vi "OpenG Dictionary.vi"() -> ()   [LabVIEW 2013]
uses:
  <userlib>/_OpenG.lib/dictionary/dictionary.llb/Dictionary Update (by scalar value)__ogtk.vi
panel:
  out "get value":variant
  in  "key":string
  in  "Get Value":bool
  out "item poped":cluster{"key":variant, "value":variant}
  in  "Pop":bool
  in  "item to be added":cluster{"key":string, "Value":dbl}
  in  "Add":bool
  out "items":cluster{"key":variant, "value":variant}[](array[cluster])
  out "Dict size":i32
  in  "stop":bool
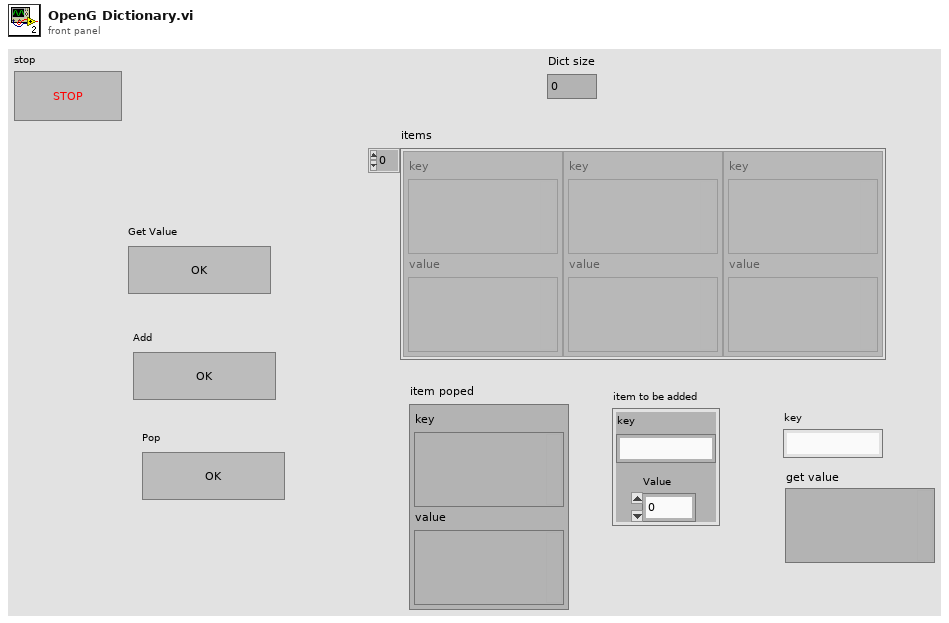
[diagram p1: front panel]
types:
  T1 = typedef "Dictionary Object RefNum__ogtk.ctl" = refnum<k1>
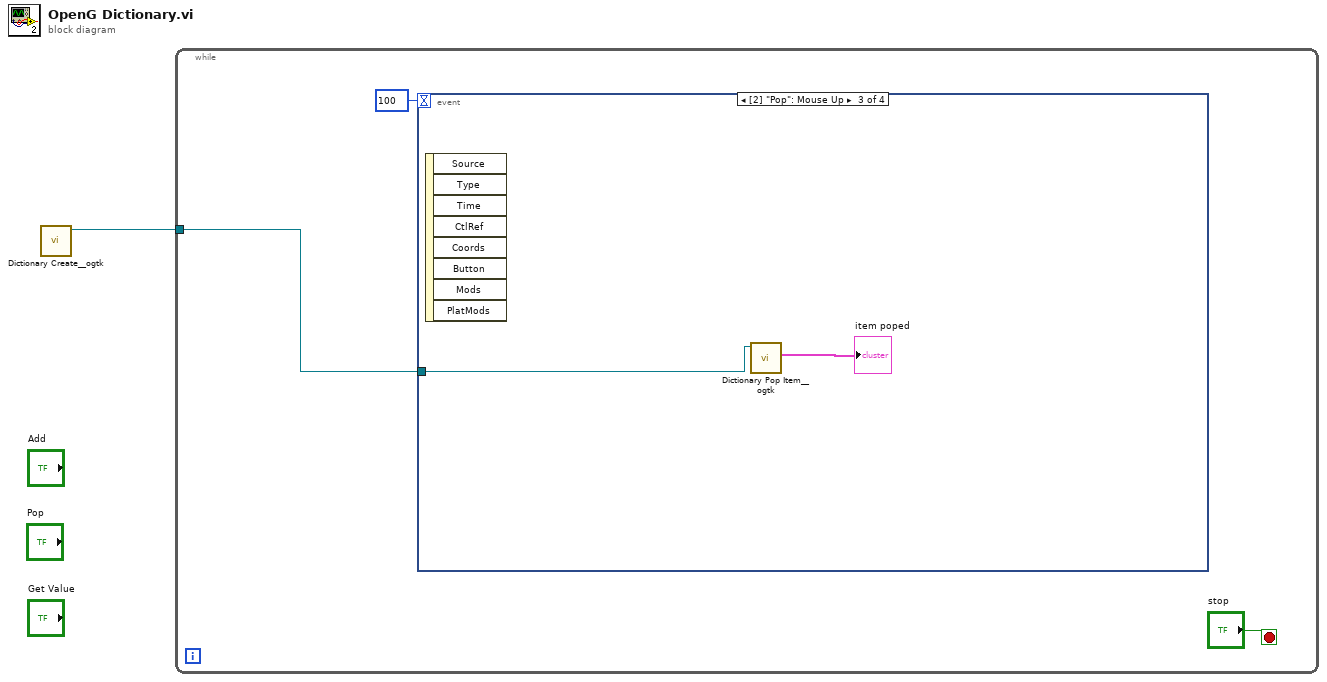
[diagram p0: block diagram]
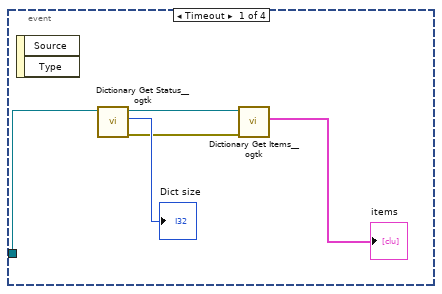
[diagram p2: hidden frame]
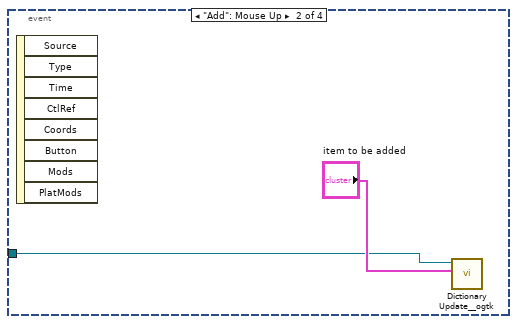
[diagram p3: hidden frame]
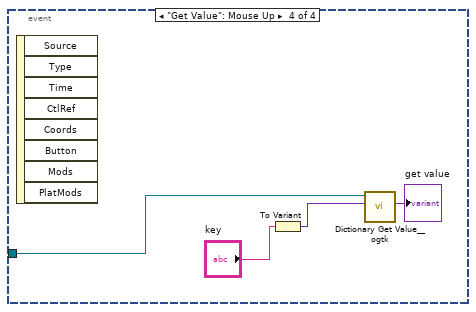
[diagram p4: hidden frame]
diagram:
  n1 = call <userlib>:"Dictionary Create__ogtk.vi"() -> ("dictionary out"=w1:T1)  [unwired: 10 in, 1 out]
  n2 = while {
    tunnel: w1 -> [w2]
    stop <- "stop" stop-if-true
    n3 = event shown="[2] \"Pop\": Mouse Up" {
      selector: _ -> [_ _ _ _]
      dyn-events: _ -> [_ _ _ _]
      timeout: 100 -> [_ _ _ _]
      tunnel: w2 -> [w9 w10 w13 w17]
      event Timeout {
        n4 = event-data() -> ()  [unwired: 1 in, 2 out]
        n5 = call <userlib>:"Dictionary Get Status__ogtk.vi"("dictionary"=w9) -> ("error out"=w6:errorcluster, "size"=→"Dict size":i32, "dictionary out"=w7:T1)  [unwired: 8 in]
        n6 = call <userlib>:"Dictionary Get Items__ogtk.vi"("error in (no error)"=w6, "dictionary"=w7) -> ("items"=→"items":cluster{"key":variant, "value":variant}[])  [unwired: 7 in, 2 out]
      }
      event "Add": Mouse Up {
        n7 = event-data() -> ()  [unwired: 1 in, 8 out]
        n8 = call-poly <userlib>:"Dictionary Update__ogtk.vi"("key-value"="item to be added", "dictionary"=w10) -> ()  [unwired: 7 in, 3 out]
      }
      event "Pop": Mouse Up {
        n9 = event-data() -> ()  [unwired: 1 in, 8 out]
        n10 = call <userlib>:"Dictionary Pop Item__ogtk.vi"("dictionary"=w13) -> ("item"=→"item poped":cluster{"key":variant, "value":variant})  [unwired: 8 in, 2 out]
      }
      event "Get Value": Mouse Up {
        n11 = event-data() -> ()  [unwired: 1 in, 8 out]
        n12 = To Variant(anything="key") -> (Variant=w15:variant)
        n13 = call <userlib>:"Dictionary Get Value__ogtk.vi"("key"=w15, "dictionary"=w17) -> ("value"=→"get value":variant)  [unwired: 6 in, 3 out]
      }
    }
  }
